vi "FPGA SPI_SPI Port.vi"(10 "Port":i8, 11 "FPGA IO":T1={"SCLK"="SCLK", "CS"="CS0", "MOSI"="MOSI", "MISO"="MISO"}) -> ()   [LabVIEW 2019]
uses:
  Controls/Port Action.ctl
  Controls/FPGA SPI_SPI Loop State.ctl
  <vilib>/Platform/TimedLoop/XDataNode/timing_clust.ctl
  <vilib>/Platform/TimedLoop/XDataNode/nitl_modes.ctl
  <vilib>/Platform/TimedLoop/XDataNode/wakeup.ctl
  <vilib>/rvi/Emulation/niFpgaGetClockAttributes.vi
  <vilib>/rvi/Emulation/niFpgaSctlEmulationGetInTimedLoop.vi
  <vilib>/rvi/Emulation/niFpgaEmulationReportErrorSimple.vi
  FPGA SPI_Globals.vi
  <vilib>/rvi/Emulation/niFpgaProcessEmulError.vi
  <vilib>/rvi/Emulation/niFpgaEmulationIsFPGAContextNoSignature.vi
  <vilib>/rvi/errors/niFpgaSetErrorForExecOnDevCompSimple.vi
  <vilib>/rvi/eio/common/nirviEmuReportErrorAndStop.vi
  <vilib>/rvi/DataTransferAndStorage/Container/Common/niFpgaContainerGetUniqueNameForEmu.vi
  <vilib>/rvi/FIFO/Fifo_Resource/nirvififoEmulationSetSize.vi
  <vilib>/rvi/FIFO/Fifo_Resource/nirviFifoEmulationQueueMgr.vi
  <instcachedir>/0/nirviFifoEmulationQueueMgr_E5CAEC123FF24DC58D834DCA3CDAA9B5.lvgen/nirviFifoEmulationQueueMgr_E5CAEC123FF24DC58D834DCA3CDAA9B5_000.vi
  <vilib>/Utility/error.llb/Clear Errors.vi
  <vilib>/rvi/FIFO/Fifo_Resource/nirvififoEmulationCreateLock.vi
  <vilib>/rvi/FIFO/Fifo_Resource/nirvififoEmulationObtainLock.vi
  <vilib>/rvi/FIFO/Fifo_Resource/nirvififoEmulationReleaseLock.vi
  <vilib>/rvi/occurrence/nirviWaitOnOccurrenceBase.vi
  <vilib>/rvi/errors/nirviReportUnexpectedCaseInternalError.vi
  <vilib>/rvi/errors/nirviReportUnexpectedCaseInternalError (U32).vi
  <vilib>/rvi/FIFO/Fifo_Resource/nirvififoEmulationDetermineInputValidOut.vi
  <vilib>/rvi/Emulation/niFpgaCriticalErrorInLSC.vi
  <vilib>/rvi/eio/common/nirviEmuTemplateMethod_errors.vi
  <vilib>/rvi/DataTransferAndStorage/Container/Common/niFpgaContainerSetEmuInfo.vi
  <vilib>/rvi/DataTransferAndStorage/Container/XNode/niFpgaContainer.xnode
  <vilib>/rvi/FIFO/Fifo_Resource/nirvififoEmulationRead.vi
  <vilib>/rvi/FIFO/Fifo_Resource/nirvififoEmulationWrite.vi
  <vilib>/Platform/TimedLoop/XDataNode/XDataNode.xnode
  <vilib>/eio/EIONode/EIONode.xnode
  <vilib>/rvi/LocalResourceManager/LocalResourceManager.xnode
  <vilib>/Platform/TimedLoop/XDataNode/XDNodeRunTimeDep.lvlib
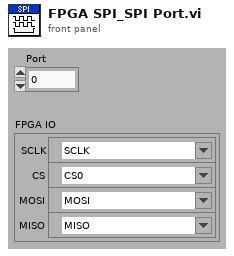
[diagram p1: front panel]
types:
  T1 = cluster{"SCLK":refnum<k21>, "CS":refnum<k21>, "MOSI":refnum<k21>, "MISO":refnum<k21>}
  T2 = cluster{"CS":u8, "CS Active State":bool, "CPOL":bool, "CPHA":bool, "Wait Ticks":u32}
  T3 = typedef "Port Action.ctl" = enum8{"Idle", "Start", "Configure Hardware", "Start Hardware", "Set Done", "Wait Until Done"}
  T4 = typedef "FPGA SPI_SPI Loop State.ctl" = enum8{"Initialize", "Read From FIFO", "Set CS", "Wait Before Set", "Set Clock", "Wait Before Reset", "Reset Clock", "Write to FIFO", "Reset CS"}
  T5 = typedef "XDNodeRunTimeDep.lvlib/timing_clust.ctl" = cluster{"Expected End [f-1]":u64, "Actual End [f-1]":u64, "Finished Late? [f-1]":bool, "Expected End [i-1]":u64, "Actual End [i-1]":u64, "Finished Late? [i-1]":bool, "Expected Start [i]":u64, "Actual Start [i]":u64, "Expected Start [f]":u64, "Actual Start [f]":u64, "Source Name":string, "Structure Name":string, "Period":i64, "Deadline":i64, "Offset":i64, "Start":i64, "Priority":i32, "Timeout":i32, "Mode":T6, "Wakeup Reason":T7, "Error":errorcluster, "Source Type":string, "Secondary Source Type":string, "Global End Time":u64, "Global Start Time":u64, "Frame Duration":u64, "Iteration Duration":u64, "Assigned CPU":i32, "I/O Scan Engine Mode":u32}
  T6 = typedef "XDNodeRunTimeDep.lvlib/nitl_modes.ctl" = enum32{"No Change", "Process missed periods, maintain original phase", "Discard missed periods, maintain original phase", "Process missed periods, ignore original phase", "Discard missed periods, ignore original phase"}
  T7 = typedef "XDNodeRunTimeDep.lvlib/wakeup.ctl" = enum32{"Normal", "Aborted", "Asynchronous wakeup", "Timing source error", "Timed loop error", "Timeout"}
  T8 = typedef "FPGA SPI_FPGA SPI State.ctl" = enum8{"Idle", "Read/Write SPI", "Configure"}
  T9 = cluster{"MOSI":bool[], "MISO":bool[], "MOSI Byte Index":i8, "MISO Byte Index":i8}
  T10 = cluster{"Next State":T4, "Wait Count":u32, "Total Bits":u16, "Current Bit":u16, "Total Bytes":u16}
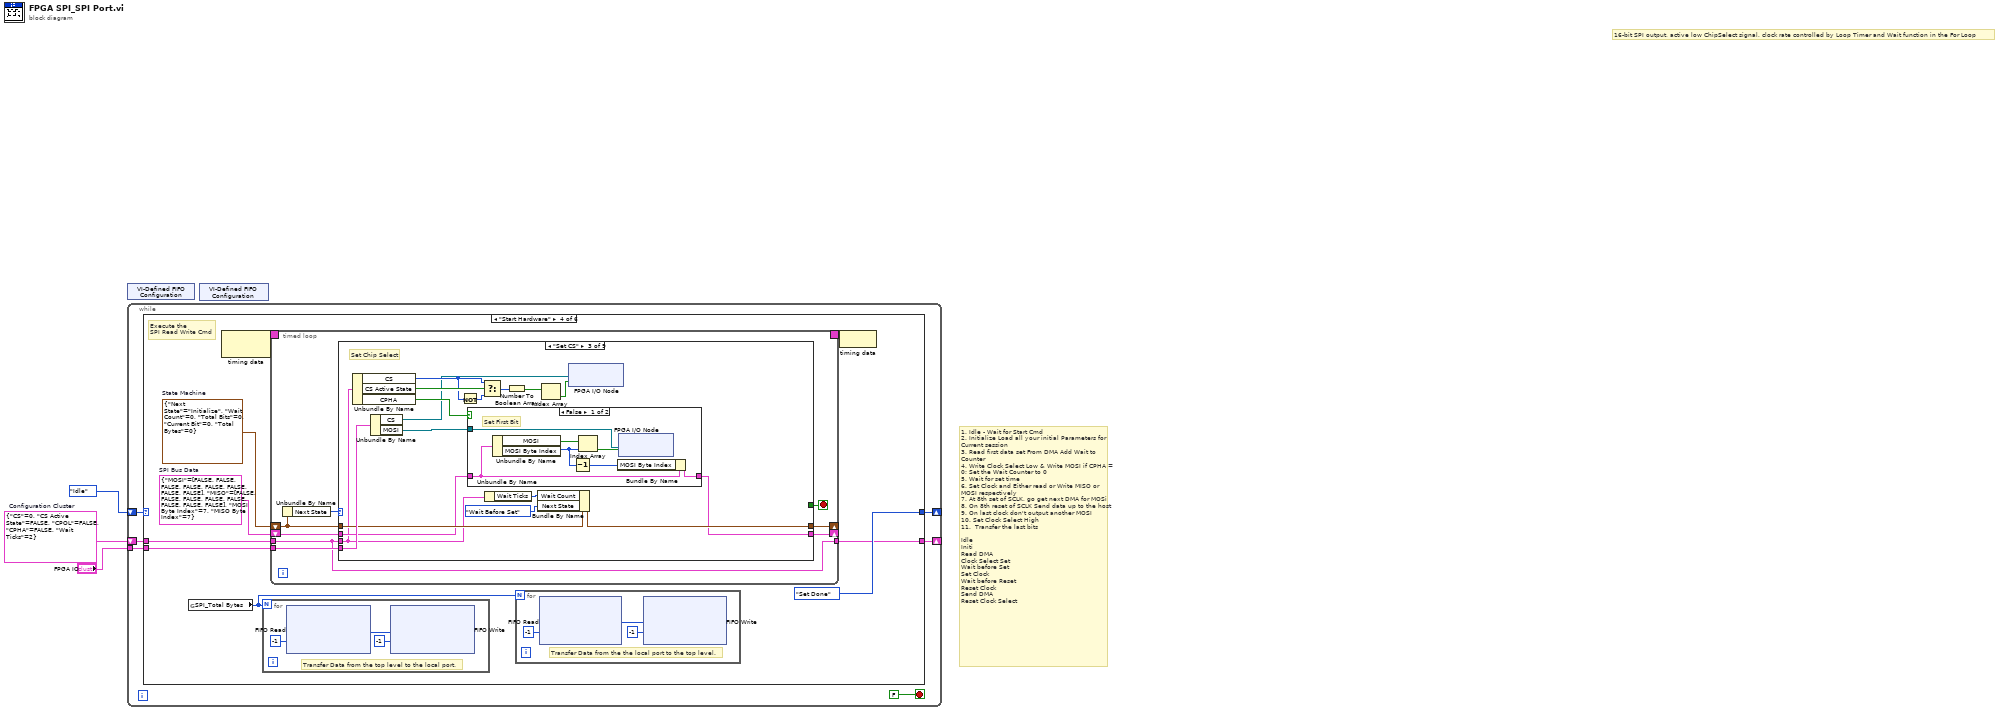
[diagram p0: block diagram]
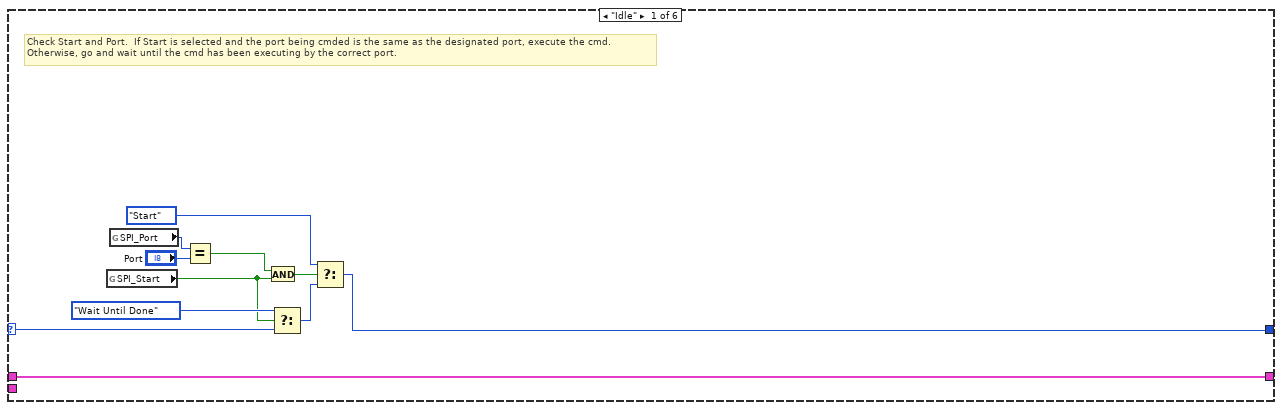
[diagram p2: hidden frame]
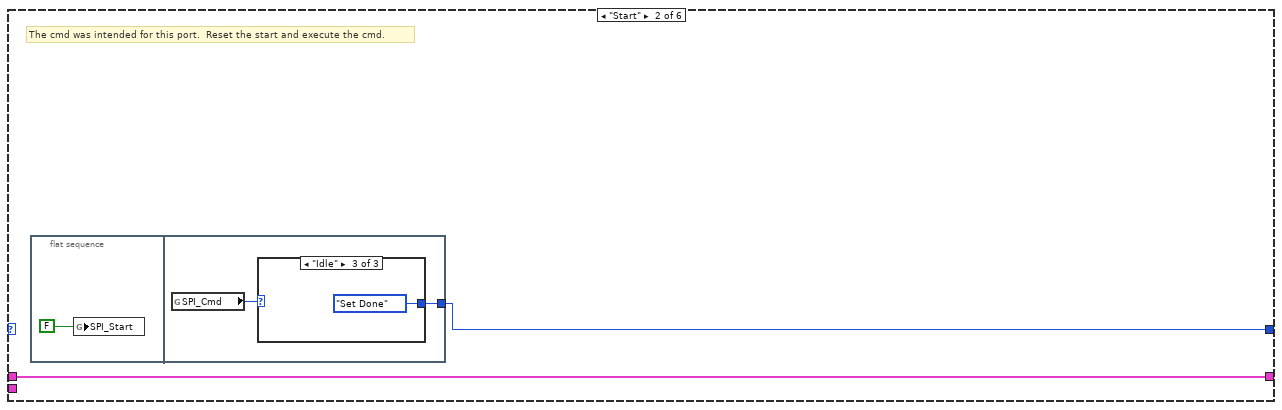
[diagram p3: hidden frame]
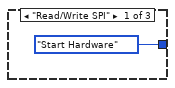
[diagram p4: hidden frame]
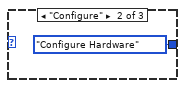
[diagram p5: hidden frame]
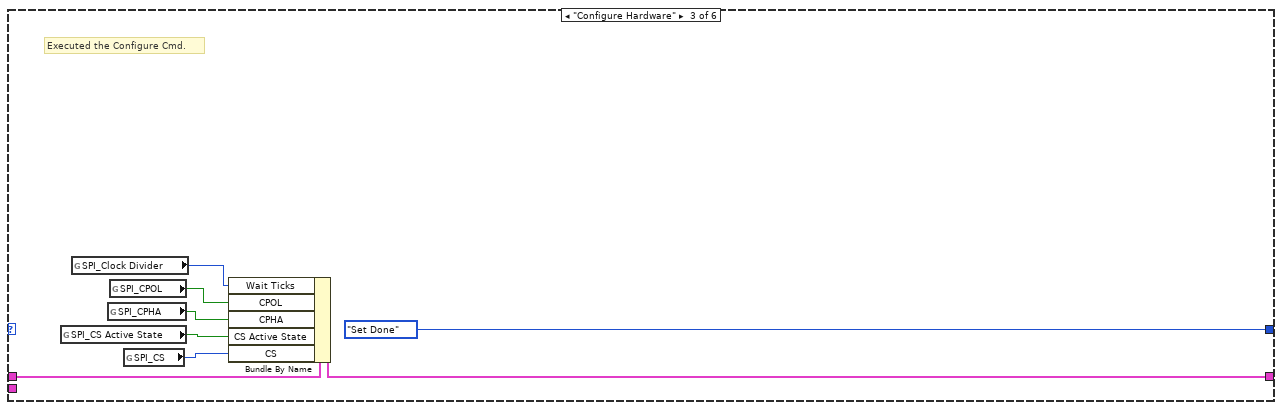
[diagram p6: hidden frame]
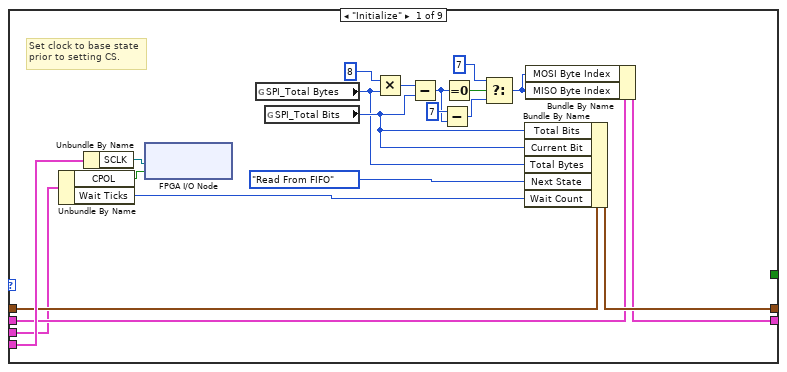
[diagram p7: hidden frame]
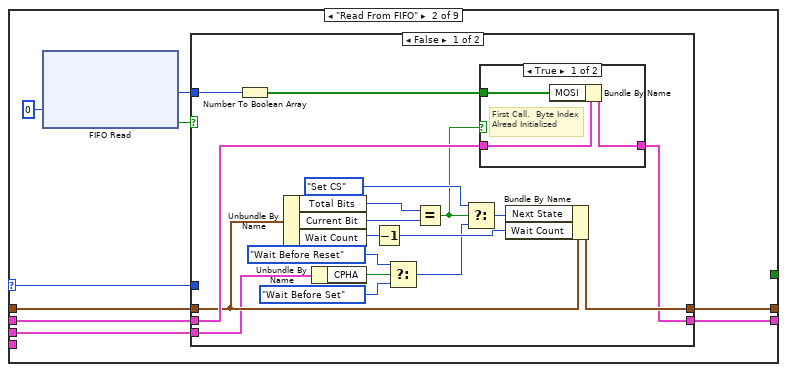
[diagram p8: hidden frame]
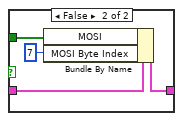
[diagram p9: hidden frame]
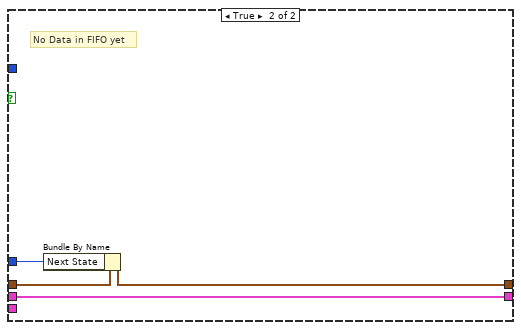
[diagram p10: hidden frame]
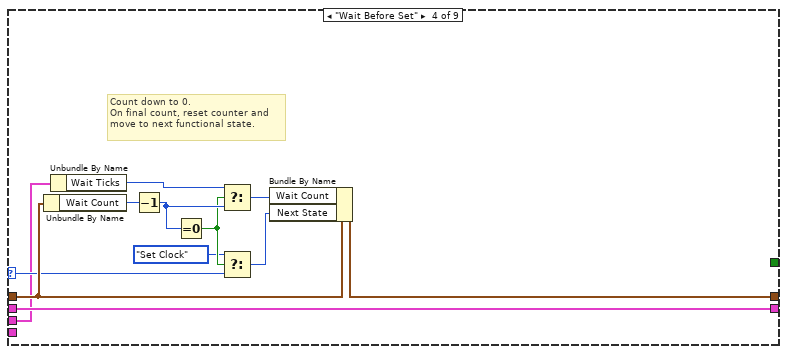
[diagram p12: hidden frame]
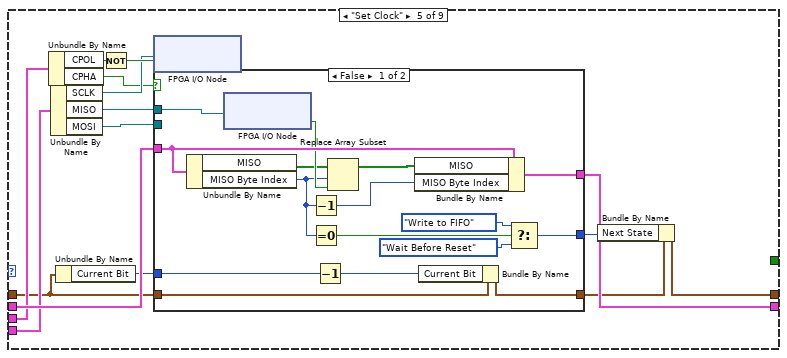
[diagram p13: hidden frame]
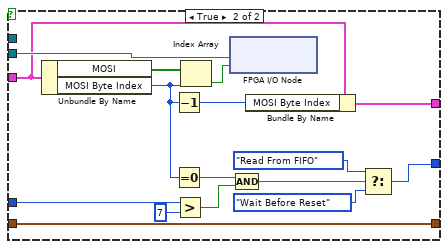
[diagram p14: hidden frame]
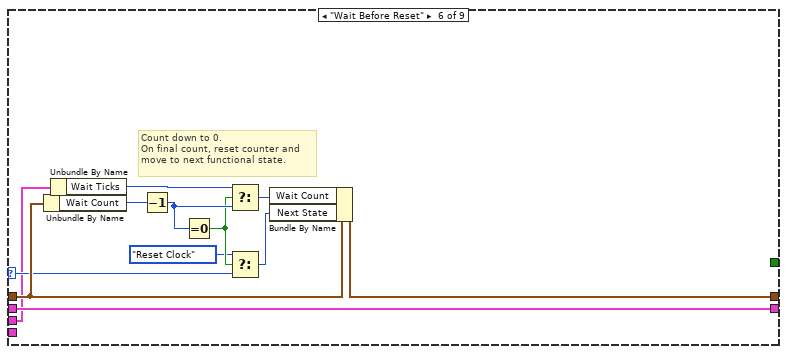
[diagram p15: hidden frame]
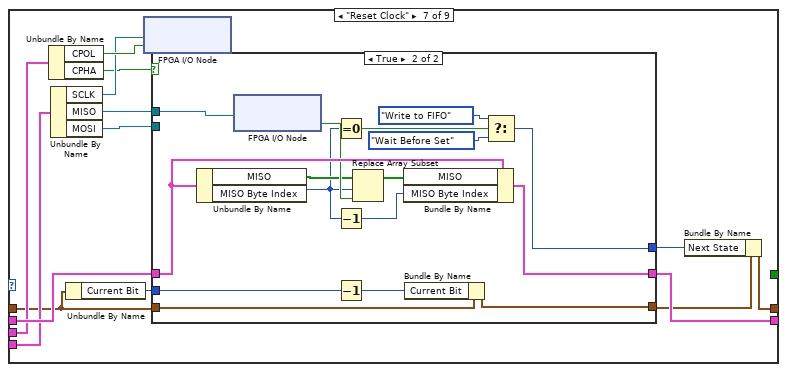
[diagram p16: hidden frame]
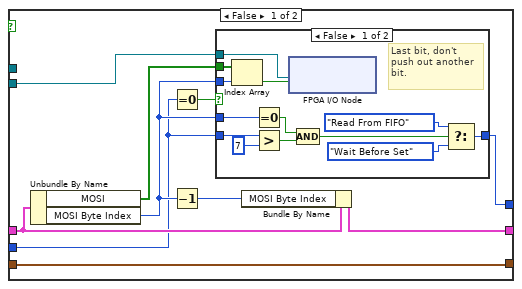
[diagram p17: hidden frame]
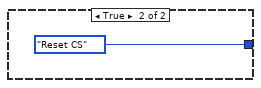
[diagram p18: hidden frame]
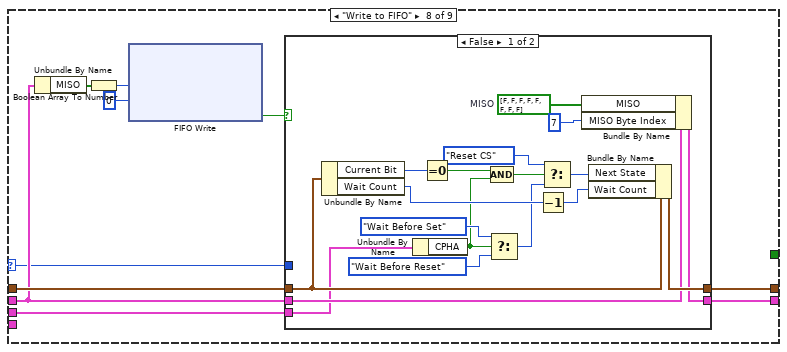
[diagram p19: hidden frame]
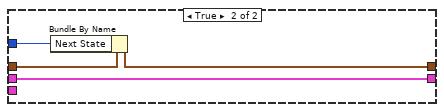
[diagram p20: hidden frame]
diagram:
  w2 = T2 {"CS"=0, "CS Active State"=FALSE, "CPOL"=FALSE, "CPHA"=FALSE, "Wait Ticks"=2}  # Configuration Cluster
  # "16-bit SPI output, active low ChipSelect signal, clock rate controlled by Loop Timer and Wait function in the For Loop"
  # "1. Idle - Wait for Start Cmd\n2. Initialize Load all your initial Parameters for Current session\n3. Read first data set From DMA Add Wait to Counter\n4. Write Clock Select Low & Write MOSI if CPHA = 0; Set the Wait Counter to 0\n5. Wait for set time\n6. Set Clock and Either read or Write MISO or MOSI respectively\n7. At 8th set of SCLK, go get next DMA for MOSi\n8. On 8th reset of SCLK Send data up to the host\n9. On last clock don't output another MOSI\n10. Set Clock Select High \n11.  Transfer the last bits\n\nIdle\nIniti\nRead DMA\nClock Select Set\nWait before Set\nSet Clock\nWait before Reset\nReset Clock\nSend DMA\nReset Clock Select"
  n1 = xnode "VI-Defined FIFO Configuration"() -> ()  [unwired: 1 out]
  n2 = while {
    shift-right: [w8] -> _
    shift-left: Port_Action."Idle" ("Action") -> [w7]
    shift-right: [w4] -> _
    shift-left: w2 -> [w6]
    tunnel: "FPGA IO" -> [w5]
    stop <- FALSE stop-if-true
    n3 = case shown="\"Start Hardware\"" w7 {
      selector: w7 -> [w10 _ _ _ _ w319]
      tunnel: [w19 w22 Port_Action."Set Done" ("Action") Port_Action."Set Done" ("Action") Port_Action."Idle" ("Action") w318] -> w8
      tunnel: w6 -> [w14 w21 w32 w37 w314 w317]
      tunnel: w5 -> [_ _ _ w42 _ _]
      tunnel: [w14 w21 w31 w38 w314 w317] -> w4
      frame "Idle" {
        # "Check Start and Port.  If Start is selected and the port being cmded is the same as the designated port, execute the cmd.\nOtherwise, go and wait until the cmd has been executing by the correct port."
        n4 = global read "FPGA SPI_Globals.vi" "SPI_Start"() -> (w11:bool)
        n5 = global read "FPGA SPI_Globals.vi" "SPI_Port"() -> (w18:i8)
        n6 = Equal?(x=w18, y="Port") -> (x = y?=w12:bool)
        n7 = And(x=w12, y=w11) -> (x .and. y?=w16:bool)
        n8 = Select(t=Port_Action."Wait Until Done" ("Action"), s=w11, f=w10) -> (s? t:f=w15:T3)
        n9 = Select(t=Port_Action."Start" ("Action"), s=w16, f=w15) -> (s? t:f=w19:T3)
      }
      frame "Start" {
        # "The cmd was intended for this port.  Reset the start and execute the cmd."
        n10 = flat-sequence {
          tunnel: [w24] -> w22
          frame #0 {
            n11 = global write "FPGA SPI_Globals.vi" "SPI_Start"(FALSE ("Write Flag")) -> ()
          }
          frame #1 {
            n12 = global read "FPGA SPI_Globals.vi" "SPI_Cmd"() -> (w25:T8)
            n13 = case shown="\"Idle\"" w25 {
              tunnel: [Port_Action."Start Hardware" ("Action") Port_Action."Configure Hardware" ("Action") Port_Action."Set Done" ("Action")] -> w24
              frame "Read/Write SPI" {
              }
              frame "Configure" {
              }
              frame "Idle" {
              }
            }
          }
        }
      }
      frame "Configure Hardware" {
        # "Executed the Configure Cmd."
        n14 = global read "FPGA SPI_Globals.vi" "SPI_CS Active State"() -> (w34:bool)
        n15 = global read "FPGA SPI_Globals.vi" "SPI_Clock Divider"() -> (w29:u32)
        n16 = global read "FPGA SPI_Globals.vi" "SPI_CPHA"() -> (w33:bool)
        n17 = global read "FPGA SPI_Globals.vi" "SPI_CPOL"() -> (w36:bool)
        n18 = global read "FPGA SPI_Globals.vi" "SPI_CS"() -> (w35:u8)
        n19 = Bundle By Name(cluster=w32, "Wait Ticks"=w29, "CPOL"=w36, "CPHA"=w33, "CS Active State"=w34, "CS"=w35) -> (w31:T2)
      }
      frame "Start Hardware" {
        w40 = T9 {"MOSI"=[FALSE, FALSE, FALSE, FALSE, FALSE, FALSE, FALSE, FALSE], "MISO"=[FALSE, FALSE, FALSE, FALSE, FALSE, FALSE, FALSE, FALSE], "MOSI Byte Index"=7, "MISO Byte Index"=7}  # SPI Bus Data
        w41 = T10 {"Next State"=enum."Initialize", "Wait Count"=0, "Total Bits"=0, "Current Bit"=0, "Total Bytes"=0}  # State Machine
        # "Execute the \nSPI Read Write Cmd"
        n20 = global read "FPGA SPI_Globals.vi" "SPI_Total Bytes"() -> (w39:u16)
        n21 = node-c288() -> (w44:T5)  [unwired: 1 out]
        n22 = for {
          N: w39 -> [_]
          # "Transfer Data from the top level to the local port."
          n23 = xnode ("FIFO Read")("Timeout"=-1) -> ("Element"=w50:u8)  [unwired: 1 in, 2 out]
          n24 = xnode ("FIFO Write")("Element"=w50, "Timeout"=-1) -> ()  [unwired: 1 in, 2 out]
        }
        n25 = timed-loop {
          timing-out: [_] -> w43
          timing: w44 -> [_]
          shift-right: [w59] -> _
          shift-left: w41 -> [w58]
          shift-right: [w55] -> _
          shift-left: w40 -> [w56]
          tunnel: w42 -> [w53]
          tunnel: [w52] -> w38
          tunnel: w37 -> [w52]
          stop <- w54 stop-if-true
          n26 = Unbundle By Name(w58) -> ("Next State"=w57:T4)
          n27 = case shown="\"Set CS\"" w57 {
            selector: w57 -> [_ w80 _ w147 _ w205 _ w268 _]
            tunnel: w58 -> [w76 w83 w127 w153 w157 w212 w215 w274 w308]
            tunnel: [w75 w86 w134 w154 w169 w213 w227 w275 w309] -> w59
            tunnel: w52 -> [w61 w82 w122 w144 w164 w203 w223 w272 w305]
            tunnel: w56 -> [w62 w84 w124 w145 w165 w210 w225 w271 w306]
            tunnel: [w65 w85 w123 w145 w166 w210 w224 w270 w306] -> w55
            tunnel: w53 -> [w79 _ w131 _ w163 _ w222 _ w303]
            tunnel: [_ _ _ _ _ _ _ _ TRUE ("Start Hardware")] -> w54
            frame "Initialize" {
              # "Set clock to base state\nprior to setting CS."
              n28 = Unbundle By Name(w61) -> ("CPOL"=w77:bool, "Wait Ticks"=w60:u32)
              n29 = Unbundle By Name(w79) -> ("SCLK"=w78:refnum<k21>)
              n30 = xnode "FPGA I/O Node"("I/O Item"=w77, "FPGA I/O In"=w78) -> ()  [unwired: 1 out]
              n31 = global read "FPGA SPI_Globals.vi" "SPI_Total Bytes"() -> (w63:u16)
              n32 = global read "FPGA SPI_Globals.vi" "SPI_Total Bits"() -> (w64:u16)
              n33 = Multiply(x=u16 8 ("y"), y=w63) -> (x*y=w72:u16)
              n34 = Subtract(x=w72, y=w64) -> (x-y=w69:i8)
              n35 = Subtract(x=i8 7, y=w69) -> (x-y=w67:i8)
              n36 = Equal To 0?(x=w69) -> (x = 0?=w68:bool)
              n37 = Select(t=i8 7 ("y"), s=w68, f=w67) -> (s? t:f=w66:i8)
              n38 = Bundle By Name(cluster=w76, "Total Bits"=w64, "Current Bit"=w64, "Total Bytes"=w63, "Next State"=FPGA_SPI_SPI_Loop_State."Read From FIFO", "Wait Count"=w60) -> (w75:T10)
              n39 = Bundle By Name(cluster=w62, "MOSI Byte Index"=w66, "MISO Byte Index"=w66) -> (w65:T9)
            }
            frame "Read From FIFO" {
              n40 = xnode ("FIFO Read")("Timeout"=0) -> ("Element"=w87:u8, "Timed Out?"=w81:bool)  [unwired: 1 in, 1 out]
              n41 = case shown="False" w81 {
                tunnel: w87 -> [w106 _]
                tunnel: [w105 w114] -> w86
                tunnel: [w100 w117] -> w85
                tunnel: w84 -> [w99 w117]
                tunnel: w83 -> [w97 w115]
                tunnel: w82 -> [w89 _]
                tunnel: w80 -> [_ w116]
                frame False {
                  n42 = Number To Boolean Array(number=w106) -> (Boolean array=w98:bool[])
                  n43 = Unbundle By Name(w97) -> ("Total Bits"=w102:u16, "Current Bit"=w104:u16, "Wait Count"=w96:u32)
                  n44 = Unbundle By Name(w89) -> ("CPHA"=w93:bool)
                  n45 = Decrement(x=w96) -> (x-1=w95:u32)
                  n46 = Select(t=FPGA_SPI_SPI_Loop_State."Wait Before Reset" ("Next State"), s=w93, f=FPGA_SPI_SPI_Loop_State."Wait Before Set" ("Next State")) -> (s? t:f=w90:T4)
                  n47 = Equal?(x=w102, y=w104) -> (x = y?=w94:bool)
                  n48 = Select(t=FPGA_SPI_SPI_Loop_State."Set CS" ("Next State"), s=w94, f=w90) -> (s? t:f=w101:T4)
                  n49 = case shown="True" w94 {
                    tunnel: [w109 w113] -> w100
                    tunnel: w99 -> [w108 w112]
                    tunnel: w98 -> [w107 w111]
                    frame True {
                      # "First Call.  Byte Index Alread Initialized"
                      n50 = Bundle By Name(cluster=w108, "MOSI"=w107) -> (w109:T9)
                    }
                    frame False {
                      n51 = Bundle By Name(cluster=w112, "MOSI"=w111, "MOSI Byte Index"=i8 7) -> (w113:T9)
                    }
                  }
                  n52 = Bundle By Name(cluster=w97, "Next State"=w101, "Wait Count"=w95) -> (w105:T10)
                }
                frame True {
                  # "No Data in FIFO yet"
                  n53 = Bundle By Name(cluster=w115, "Next State"=w116) -> (w114:T10)
                }
              }
            }
            frame "Set CS" {
              # "Set Chip Select"
              n54 = Unbundle By Name(w122) -> ("CS"=w128:u8, "CS Active State"=w133:bool, "CPHA"=w129:bool)
              n55 = Unbundle By Name(w131) -> ("CS"=w121:refnum<k21>, "MOSI"=w130:refnum<k21>)
              n56 = Not(x=w128) -> (.not. x?=w132:u8)
              n57 = case shown="False" w129 {
                tunnel: w124 -> [w137 w142]
                tunnel: w130 -> [w139 _]
                tunnel: [w135 w142] -> w123
                frame False {
                  # "Set First Bit"
                  n58 = Unbundle By Name(w137) -> ("MOSI"=w141:bool[], "MOSI Byte Index"=w138:i8)
                  n59 = Decrement(x=w138) -> (x-1=w136:i8)
                  n60 = Index Array(array=w141, index=w138) -> (element=w140:bool)
                  n61 = Bundle By Name(cluster=w137, "MOSI Byte Index"=w136) -> (w135:T9)
                  n62 = xnode "FPGA I/O Node"("I/O Item"=w140, "FPGA I/O In"=w139) -> ()  [unwired: 1 out]
                }
                frame True {
                }
              }
              n63 = Select(t=w128, s=w133, f=w132) -> (s? t:f=w119:u8)
              n64 = Unbundle By Name(w122) -> ("Wait Ticks"=w126:u32)
              n65 = Number To Boolean Array(number=w119) -> (Boolean array=w120:bool[])
              n66 = Bundle By Name(cluster=w127, "Wait Count"=w126, "Next State"=FPGA_SPI_SPI_Loop_State."Wait Before Set" ("Enum")) -> (w134:T10)
              n67 = Index Array(array=w120) -> (element=w118:bool)  [unwired: 1 in]
              n68 = xnode "FPGA I/O Node"("I/O Item"=w118, "FPGA I/O In"=w121) -> ()  [unwired: 1 out]
            }
            frame "Wait Before Set" {
              # "Count down to 0.\nOn final count, reset counter and\nmove to next functional state."
              n69 = Unbundle By Name(w153) -> ("Wait Count"=w151:u32)
              n70 = Unbundle By Name(w144) -> ("Wait Ticks"=w143:u32)
              n71 = Decrement(x=w151) -> (x-1=w152:u32)
              n72 = Equal To 0?(x=w152) -> (x = 0?=w150:bool)
              n73 = Select(t=w143, s=w150, f=w152) -> (s? t:f=w149:u32)
              n74 = Select(t=FPGA_SPI_SPI_Loop_State."Set Clock", s=w150, f=w147) -> (s? t:f=w148:T4)
              n75 = Bundle By Name(cluster=w153, "Wait Count"=w149, "Next State"=w148) -> (w154:T10)
            }
            frame "Set Clock" {
              n76 = Unbundle By Name(w164) -> ("CPOL"=w167:bool, "CPHA"=w159:bool)
              n77 = Unbundle By Name(w163) -> ("SCLK"=w160:refnum<k21>, "MISO"=w161:refnum<k21>, "MOSI"=w162:refnum<k21>)
              n78 = Unbundle By Name(w157) -> ("Current Bit"=w156:u16)
              n79 = Not(x=w167) -> (.not. x?=w168:bool)
              n80 = xnode "FPGA I/O Node"("I/O Item"=w168, "FPGA I/O In"=w160) -> ()  [unwired: 1 out]
              n81 = case shown="False" w159 {
                tunnel: [w185 w188] -> w166
                tunnel: w165 -> [w184 w189]
                tunnel: w162 -> [_ w199]
                tunnel: w161 -> [w179 _]
                tunnel: w157 -> [w178 w198]
                tunnel: [w177 w198] -> w158
                tunnel: w156 -> [w176 w196]
                tunnel: [w171 w190] -> w155
                frame False {
                  n82 = Unbundle By Name(w184) -> ("MISO"=w182:bool[], "MISO Byte Index"=w175:i8)
                  n83 = xnode "FPGA I/O Node"("FPGA I/O In"=w179) -> ("I/O Item"=w183:bool)  [unwired: 1 out]
                  n84 = Decrement(x=w175) -> (x-1=w180:i8)
                  n85 = Equal To 0?(x=w175) -> (x = 0?=w170:bool)
                  n86 = Decrement(x=w176) -> (x-1=w174:u16)
                  n87 = Replace Array Subset(array=w182, new element=w183, index=w175) -> (w181:bool[])
                  n88 = Bundle By Name(cluster=w184, "MISO"=w181, "MISO Byte Index"=w180) -> (w185:T9)
                  n89 = Bundle By Name(cluster=w178, "Current Bit"=w174) -> (w177:T10)
                  n90 = Select(t=FPGA_SPI_SPI_Loop_State."Write to FIFO" ("Enum"), s=w170, f=FPGA_SPI_SPI_Loop_State."Wait Before Reset" ("Enum")) -> (s? t:f=w171:T4)
                }
                frame True {
                  n91 = Unbundle By Name(w189) -> ("MOSI"=w201:bool[], "MOSI Byte Index"=w187:i8)
                  n92 = Decrement(x=w187) -> (x-1=w186:i8)
                  n93 = Equal To 0?(x=w187) -> (x = 0?=w197:bool)
                  n94 = Greater?(x=w196, y=u16 7 ("x")) -> (0:w194:bool)
                  n95 = Index Array(array=w201, index=w187) -> (element=w200:bool)
                  n96 = xnode "FPGA I/O Node"("I/O Item"=w200, "FPGA I/O In"=w199) -> ()  [unwired: 1 out]
                  n97 = Compound Arithmetic op=AND(w197, w194) -> (w193:bool)
                  n98 = Bundle By Name(cluster=w189, "MOSI Byte Index"=w186) -> (w188:T9)
                  n99 = Select(t=FPGA_SPI_SPI_Loop_State."Read From FIFO" ("Enum"), s=w193, f=FPGA_SPI_SPI_Loop_State."Wait Before Reset" ("Enum")) -> (s? t:f=w190:T4)
                }
              }
              n100 = Bundle By Name(cluster=w158, "Next State"=w155) -> (w169:T10)
            }
            frame "Wait Before Reset" {
              # "Count down to 0.\nOn final count, reset counter and\nmove to next functional state."
              n101 = Unbundle By Name(w212) -> ("Wait Count"=w209:u32)
              n102 = Unbundle By Name(w203) -> ("Wait Ticks"=w202:u32)
              n103 = Decrement(x=w209) -> (x-1=w211:u32)
              n104 = Equal To 0?(x=w211) -> (x = 0?=w208:bool)
              n105 = Select(t=w202, s=w208, f=w211) -> (s? t:f=w207:u32)
              n106 = Select(t=FPGA_SPI_SPI_Loop_State."Reset Clock", s=w208, f=w205) -> (s? t:f=w206:T4)
              n107 = Bundle By Name(cluster=w212, "Wait Count"=w207, "Next State"=w206) -> (w213:T10)
            }
            frame "Reset Clock" {
              n108 = Unbundle By Name(w223) -> ("CPOL"=w226:bool, "CPHA"=w218:bool)
              n109 = Unbundle By Name(w222) -> ("SCLK"=w219:refnum<k21>, "MISO"=w220:refnum<k21>, "MOSI"=w221:refnum<k21>)
              n110 = Unbundle By Name(w215) -> ("Current Bit"=w214:u16)
              n111 = xnode "FPGA I/O Node"("I/O Item"=w226, "FPGA I/O In"=w219) -> ()  [unwired: 1 out]
              n112 = case shown="True" w218 {
                tunnel: [w232 w263] -> w224
                tunnel: w225 -> [w233 w267]
                tunnel: w221 -> [w237 _]
                tunnel: w220 -> [_ w264]
                tunnel: w215 -> [w234 w261]
                tunnel: [w234 w260] -> w217
                tunnel: [w228 w254] -> w216
                tunnel: w214 -> [w229 w252]
                frame False {
                  n113 = Unbundle By Name(w233) -> ("MOSI"=w236:bool[], "MOSI Byte Index"=w230:i8)
                  n114 = Equal To 0?(x=w229) -> (x = 0?=w235:bool)
                  n115 = Decrement(x=w230) -> (x-1=w231:i8)
                  n116 = case shown="False" w235 {
                    tunnel: w237 -> [w249 _]
                    tunnel: w236 -> [w248 _]
                    tunnel: w230 -> [w247 _]
                    tunnel: w230 -> [w243 _]
                    tunnel: w229 -> [w242 _]
                    tunnel: [w238 FPGA_SPI_SPI_Loop_State."Reset CS" ("Enum")] -> w228
                    frame False {
                      # "Last bit, don't\npush out another\nbit."
                      n117 = Index Array(array=w248, index=w247) -> (element=w250:bool)
                      n118 = Equal To 0?(x=w243) -> (x = 0?=w245:bool)
                      n119 = Greater?(x=w242, y=u16 7 ("x")) -> (0:w246:bool)
                      n120 = xnode "FPGA I/O Node"("I/O Item"=w250, "FPGA I/O In"=w249) -> ()  [unwired: 1 out]
                      n121 = Compound Arithmetic op=AND(w245, w246) -> (w239:bool)
                      n122 = Select(t=FPGA_SPI_SPI_Loop_State."Read From FIFO" ("Enum"), s=w239, f=FPGA_SPI_SPI_Loop_State."Wait Before Set" ("Enum")) -> (s? t:f=w238:T4)
                    }
                    frame True {
                    }
                  }
                  n123 = Bundle By Name(cluster=w233, "MOSI Byte Index"=w231) -> (w232:T9)
                }
                frame True {
                  n124 = Unbundle By Name(w267) -> ("MISO"=w265:bool[], "MISO Byte Index"=w256:i8)
                  n125 = xnode "FPGA I/O Node"("FPGA I/O In"=w264) -> ("I/O Item"=w266:bool)  [unwired: 1 out]
                  n126 = Equal To 0?(x=w256) -> (x = 0?=w253:bool)
                  n127 = Decrement(x=w256) -> (x-1=w259:i8)
                  n128 = Decrement(x=w252) -> (x-1=w255:u16)
                  n129 = Replace Array Subset(array=w265, new element=w266, index=w256) -> (w262:bool[])
                  n130 = Bundle By Name(cluster=w267, "MISO"=w262, "MISO Byte Index"=w259) -> (w263:T9)
                  n131 = Bundle By Name(cluster=w261, "Current Bit"=w255) -> (w260:T10)
                  n132 = Select(t=FPGA_SPI_SPI_Loop_State."Write to FIFO" ("Enum"), s=w253, f=FPGA_SPI_SPI_Loop_State."Wait Before Set" ("Enum")) -> (s? t:f=w254:T4)
                }
              }
              n133 = Bundle By Name(cluster=w217, "Next State"=w216) -> (w227:T10)
            }
            frame "Write to FIFO" {
              n134 = Unbundle By Name(w271) -> ("MISO"=w277:bool[])
              n135 = Boolean Array To Number(Boolean array=w277) -> (number=w276:u8)
              n136 = xnode ("FIFO Write")("Element"=w276, "Timeout"=0) -> ("Timed Out?"=w269:bool)  [unwired: 1 in, 1 out]
              n137 = case shown="False" w269 {
                tunnel: [w295 w297] -> w275
                tunnel: w274 -> [w294 w298]
                tunnel: w272 -> [w278 _]
                tunnel: w271 -> [w281 w299]
                tunnel: [w279 w299] -> w270
                tunnel: w268 -> [_ w296]
                frame False {
                  w282 = bool[] [FALSE, FALSE, FALSE, FALSE, FALSE, FALSE, FALSE, FALSE]  # MISO
                  n138 = Unbundle By Name(w294) -> ("Current Bit"=w293:u16, "Wait Count"=w290:u32)
                  n139 = Unbundle By Name(w278) -> ("CPHA"=w284:bool)
                  n140 = Equal To 0?(x=w293) -> (x = 0?=w286:bool)
                  n141 = Select(t=FPGA_SPI_SPI_Loop_State."Wait Before Set" ("Next State"), s=w284, f=FPGA_SPI_SPI_Loop_State."Wait Before Reset" ("Next State")) -> (s? t:f=w287:T4)
                  n142 = Compound Arithmetic op=AND(w286, w284) -> (w285:bool)
                  n143 = Decrement(x=w290) -> (x-1=w283:u32)
                  n144 = Select(t=FPGA_SPI_SPI_Loop_State."Reset CS" ("Next State"), s=w285, f=w287) -> (s? t:f=w291:T4)
                  n145 = Bundle By Name(cluster=w281, "MISO"=w282, "MISO Byte Index"=i8 7) -> (w279:T9)
                  n146 = Bundle By Name(cluster=w294, "Next State"=w291, "Wait Count"=w283) -> (w295:T10)
                }
                frame True {
                  n147 = Bundle By Name(cluster=w298, "Next State"=w296) -> (w297:T10)
                }
              }
            }
            frame "Reset CS" {
              # "Reset all CS signals.  Stop the loop."
              n148 = Unbundle By Name(w305) -> ("CS Active State"=w304:bool)
              n149 = Unbundle By Name(w303) -> ("CS"=w302:refnum<k21>)
              n150 = Not(x=w304) -> (.not. x?=w300:bool)
              n151 = Bundle By Name(cluster=w308, "Next State"=FPGA_SPI_SPI_Loop_State."Initialize" ("Enum")) -> (w309:T10)
              n152 = xnode "FPGA I/O Node"("I/O Item"=w300, "FPGA I/O In"=w302) -> ()  [unwired: 1 out]
            }
          }
        }
        n153 = for {
          N: w39 -> [_]
          # "Transfer Data from the the local port to the top level."
          n154 = xnode ("FIFO Read")("Timeout"=-1) -> ("Element"=w47:u8)  [unwired: 1 in, 2 out]
          n155 = xnode ("FIFO Write")("Element"=w47, "Timeout"=-1) -> ()  [unwired: 1 in, 2 out]
        }
        n156 = node-c288(w43) -> ()
      }
      frame "Set Done" {
        # "Set the done flag"
        n157 = global write "FPGA SPI_Globals.vi" "SPI_Done"(TRUE ("Done")) -> ()
      }
      frame "Wait Until Done" {
        # "Wait until the executing port finishes."
        n158 = global read "FPGA SPI_Globals.vi" "SPI_Done"() -> (w321:bool)
        n159 = Select(t=Port_Action."Idle" ("Action"), s=w321, f=w319) -> (s? t:f=w318:T3)
      }
    }
  }
  n160 = xnode "VI-Defined FIFO Configuration"() -> ()  [unwired: 1 out]
